vi "get data test.vi"() -> ()   [LabVIEW 2014]
uses:
  Robot Global Data.vi
panel:
  out "unsigned byte array":u8[](array[numeric])
  out "Bytes at Port":u32
  in  "Numeric 4":i32
  in  "milliseconds to wait 2":u32
  in  "milliseconds to wait":u32
  out "Received Data 7":u8[][](array[numeric])
  out "Received Data 6":u8[][](array[numeric])
  in  "write and read":bool
  in  "Numeric 3":i32
  out "Received Data 5":u8[][](array[numeric])
  in  "Numeric 2":i32
  in  "read forloop":bool=TRUE
  out "Received Data 4":u8[](array[numeric])
  in  "array input":bool
  in  "for loop":bool
  out "Received Data 3":u8[][](array[numeric])
  in  "Numeric":i32
  out "Received Data 2":u8[](array[numeric])
  out "distance 2":fxp<+/-,32,16>[](array[numeric])
  out "Received Data":u8[](array[numeric])
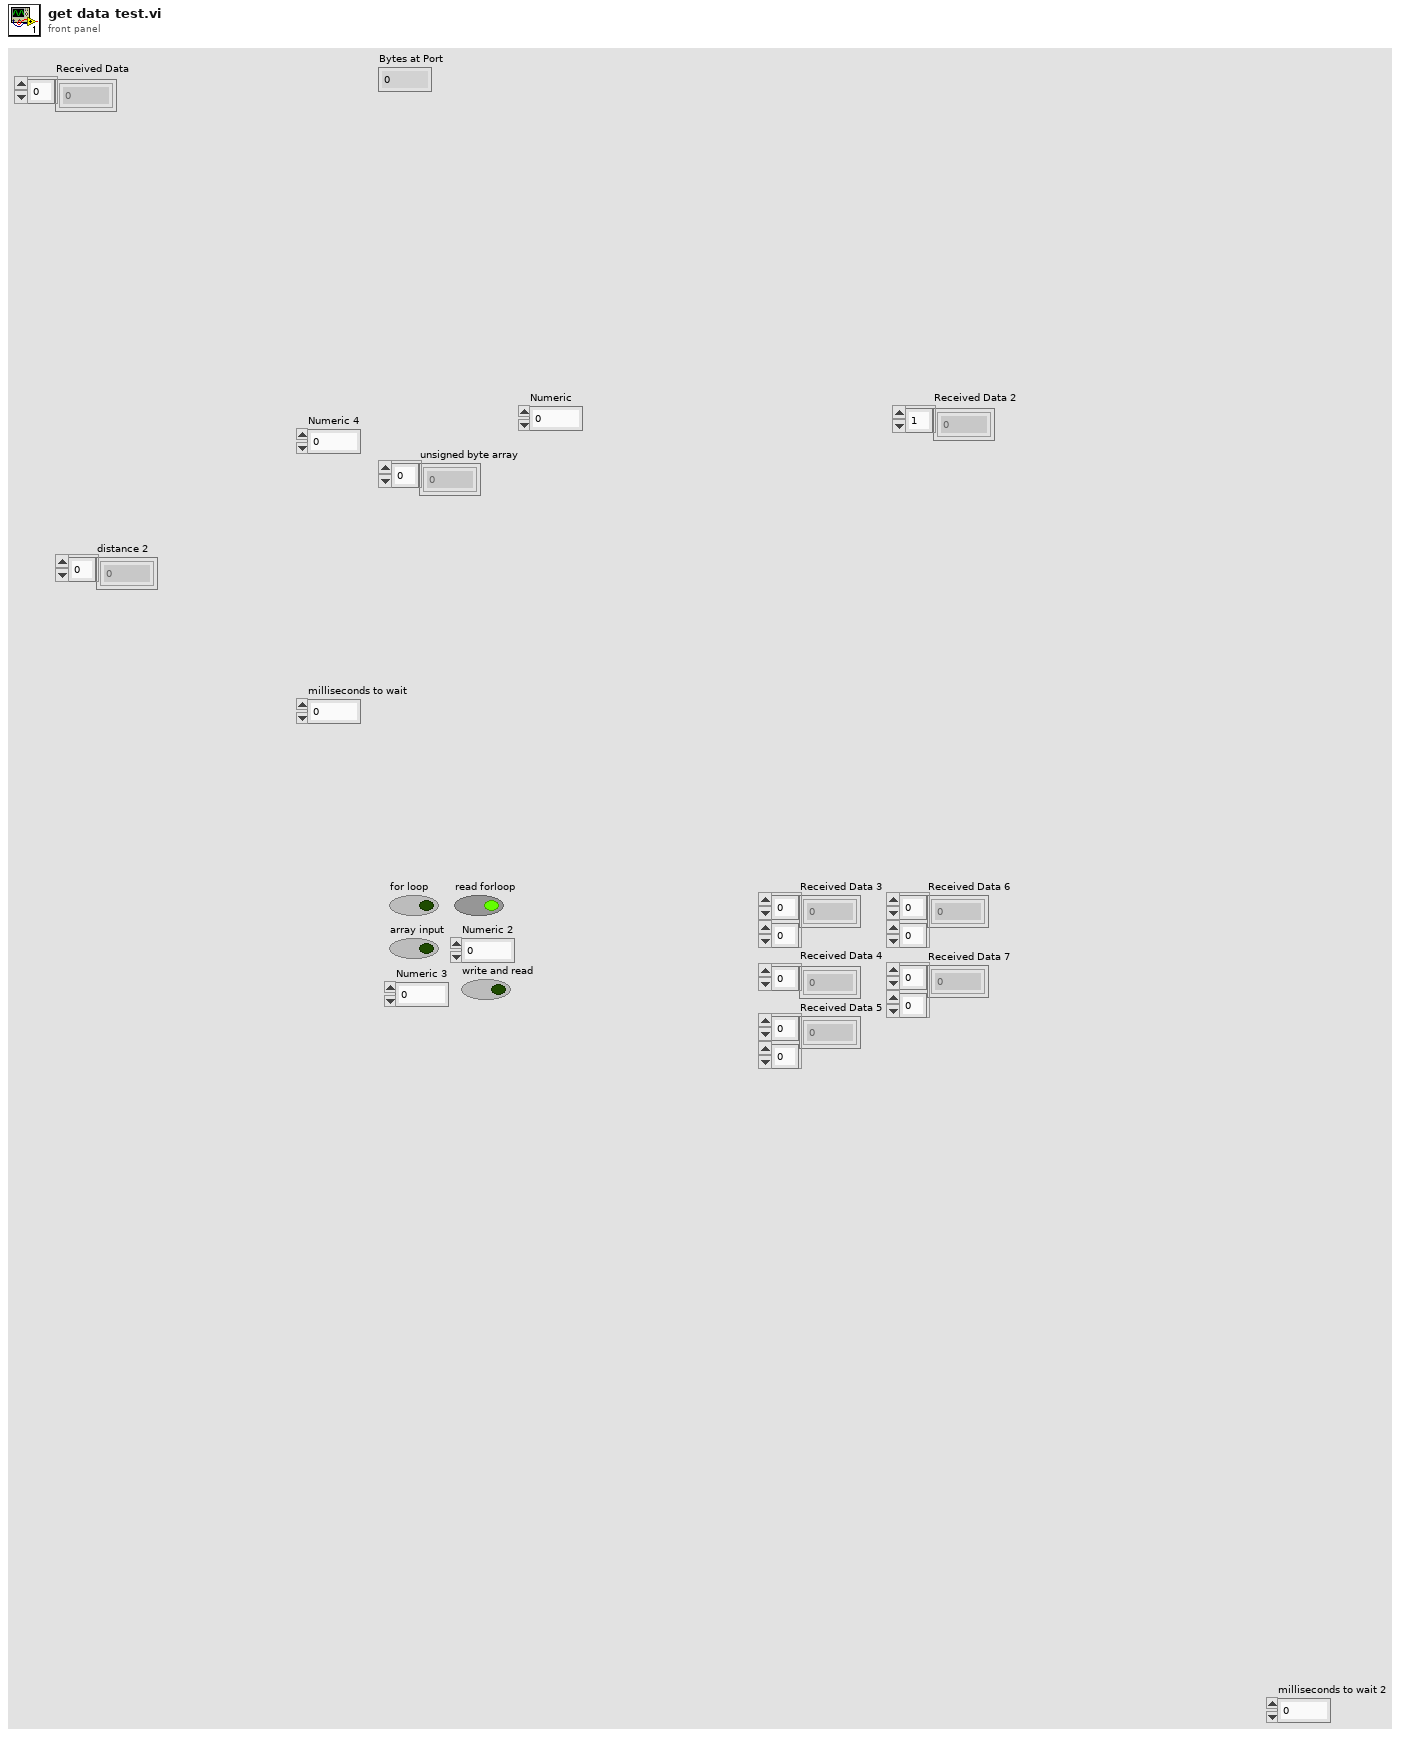
[diagram p1: front panel]
types:
  T1 = typedef "WPI_SPIDevRef.ctl" = cluster{"DevStatus":errorcluster, "Handle":i32, "Controller":T2, "SPI Bus":T3}
  T2 = typedef "FPGA_TypedefDigitalModule.ctl" = enum16{"Controller 1"}
  T3 = typedef "spi_bus.ctl" = enum16{"SPI On-Board, CS0", "SPI On-Board, CS1", "SPI On-Board, CS2", "SPI On-Board, CS3", "SPI MXP", "Invalid"}
  T4 = typedef "WPI_SerialPortRef.ctl" = cluster{"DevStatus":errorcluster, "Serial Port Name":refnum<visa-resource-name>}
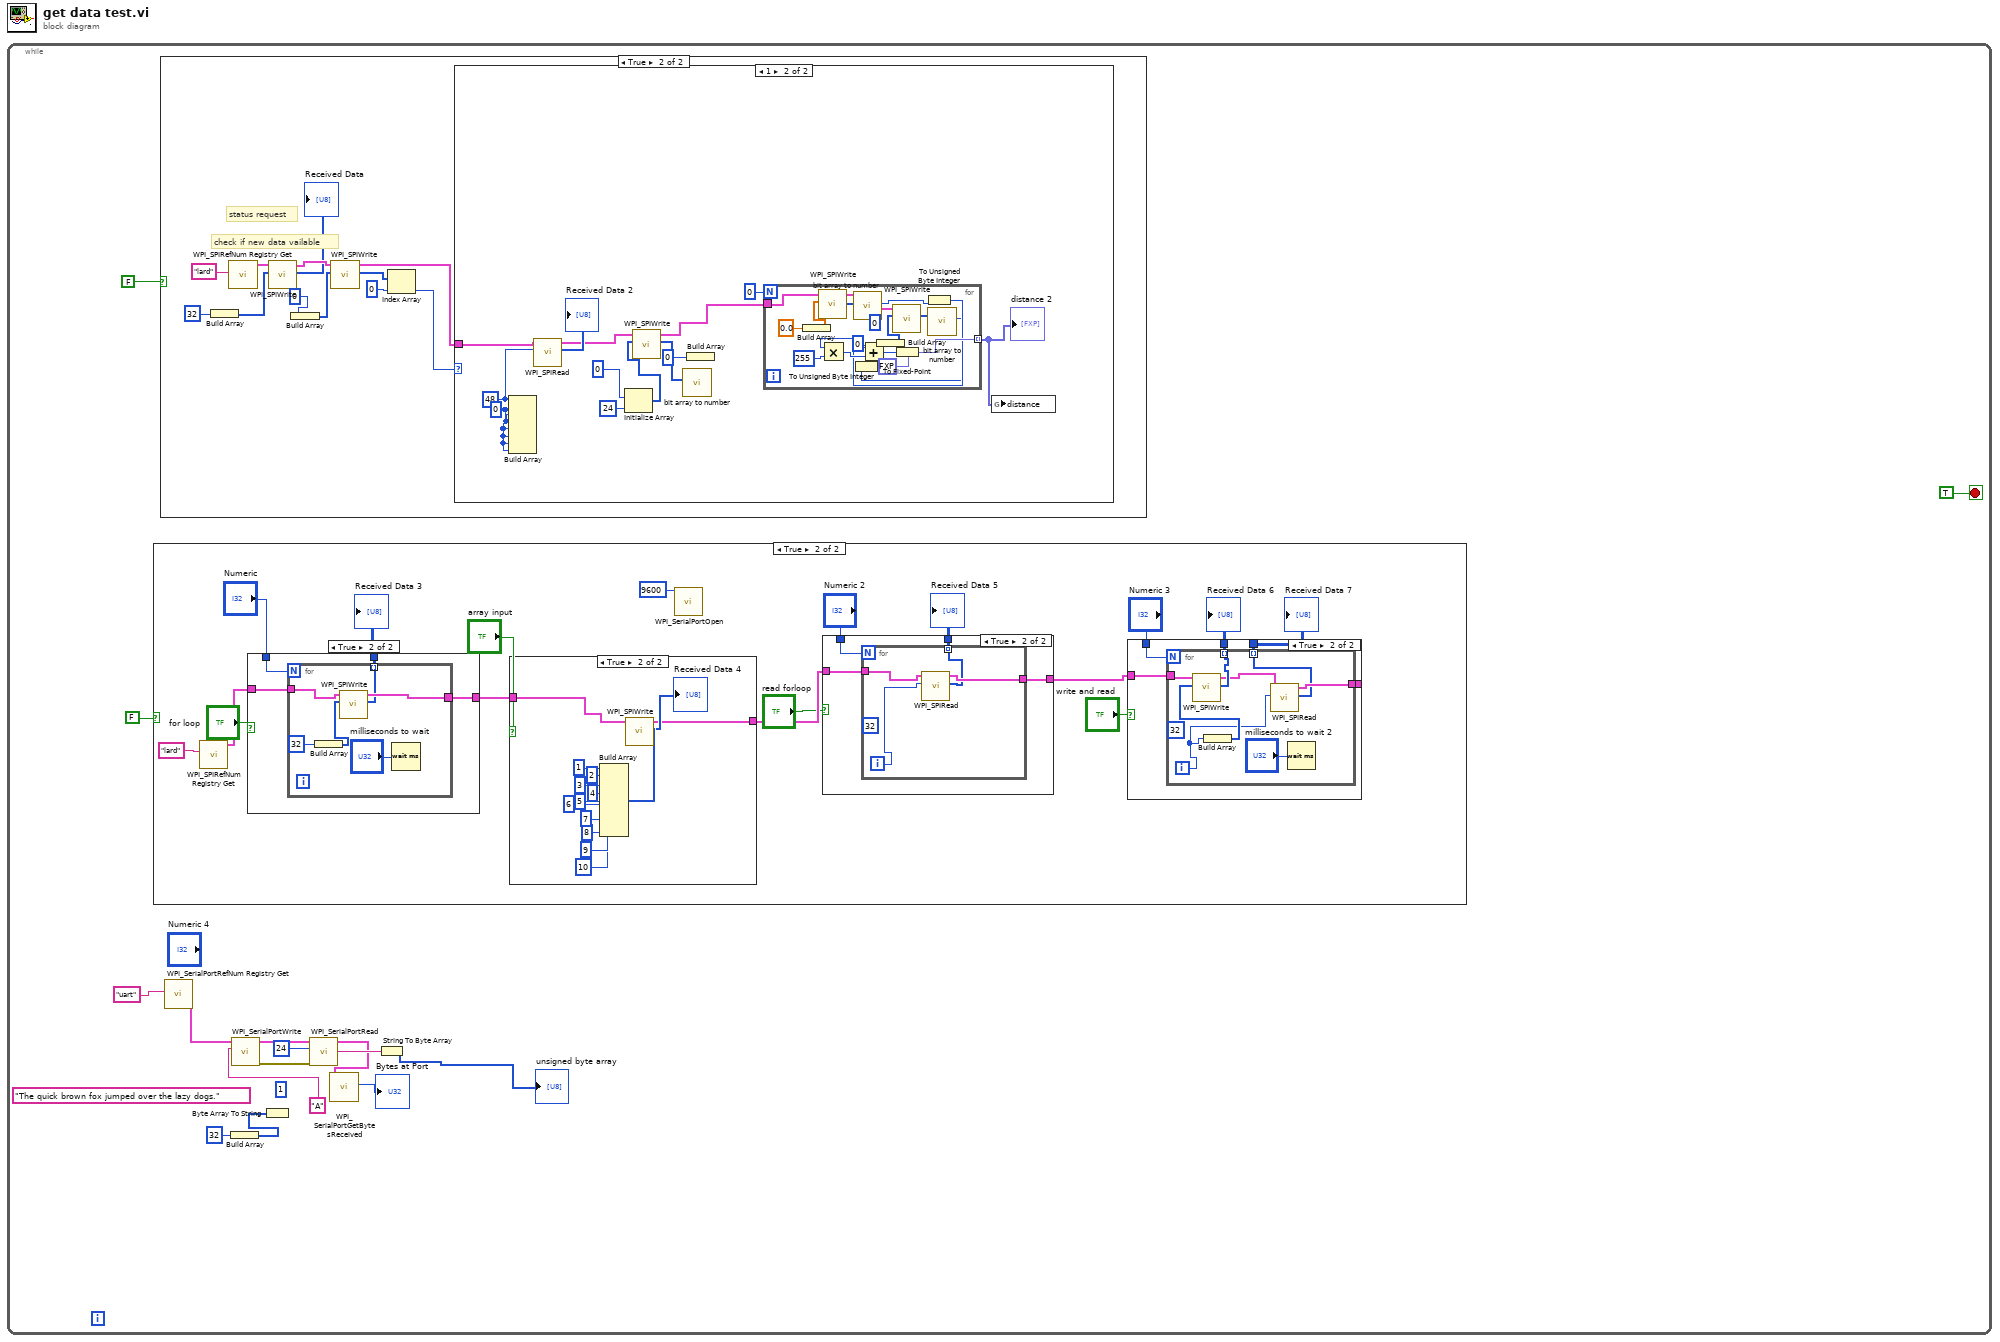
[diagram p0: block diagram]
diagram:
  n1 = while {
    stop <- TRUE stop-if-true
    (unwired) "The quick brown fox jumped over the lazy dogs." ("Buffer")
    (unwired) u32 1 ("Num Bytes to Read")
    n2 = case shown="True" FALSE {
      frame False {
      }
      frame True {
        n3 = call <vilib>:"WPI_SPIRefNum Registry Get.vi"("refnum name"="lard") -> ("SPIDevRef"=w31:T1)  [unwired: 9 in, 1 out]
        n4 = case shown="True" "for loop" {
          tunnel: w31 -> [w71 w75]
          tunnel: "Numeric" -> [_ w74]
          tunnel: [_ w73] -> w29
          tunnel: [w71 w72] -> w26
          frame False {
          }
          frame True {
            n5 = for {
              N: w74 -> [_]
              tunnel: w75 -> [w80]
              tunnel: [w78] -> w73 mode=indexing
              tunnel: [w79] -> w72
              n6 = Build Array(u8 32) -> (w77:u8[])
              n7 = call <vilib>:"WPI_SPIWrite.vi"("Data To Send"=w77, "SPIDevRef"=w80) -> ("Received Data"=w78:u8[], "SPIDevRef"=w79:T1)  [unwired: 1 in, 7 out]
              n8 = Wait (ms)(milliseconds to wait="milliseconds to wait") -> ()  [unwired: 1 out]
            }
          }
        }
        "Received Data 3" <- w29
        n9 = case shown="True" "array input" {
          tunnel: w26 -> [w56 w67]
          tunnel: [w56 w61] -> w25
          frame False {
          }
          frame True {
            n10 = Build Array(1, 2 ("element"), 3 ("element"), 4 ("element"), 5 ("element"), 6 ("element"), 7 ("element"), 8 ("element"), 9 ("element"), 10 ("element")) -> (w70:i32[])
            n11 = call <vilib>:"WPI_SPIWrite.vi"("Data To Send"=w70, "SPIDevRef"=w67) -> ("Received Data"=→"Received Data 4":u8[], "SPIDevRef"=w61:T1)  [unwired: 7 in, 1 out]
          }
        }
        n12 = call <vilib>:"WPI_SerialPortOpen.vi"("Baud Rate"=u32 9600) -> ()  [unwired: 13 in, 2 out]
        n13 = case shown="True" "read forloop" {
          tunnel: w25 -> [w47 w51]
          tunnel: "Numeric 2" -> [_ w50]
          tunnel: [_ w49] -> w22
          tunnel: [w47 w48] -> w21
          frame False {
          }
          frame True {
            n14 = for {
              N: w50 -> [_]
              tunnel: w51 -> [w55]
              tunnel: [w53] -> w49 mode=indexing
              tunnel: [w54] -> w48
              i -> [w52]
              (unwired) 32
              n15 = call <vilib>:"WPI_SPIRead.vi"("Num to Read"=w52, "SPIDevRef"=w55) -> ("Received Data"=w53:u8[], "SPIDevRef"=w54:T1)  [unwired: 1 in, 7 out]
            }
          }
        }
        "Received Data 5" <- w22
        n16 = case shown="True" "write and read" {
          tunnel: w21 -> [w33 w38]
          tunnel: "Numeric 3" -> [_ w37]
          tunnel: [_ w36] -> w17
          tunnel: [w33 w35] -> _
          tunnel: [_ w34] -> w18
          frame False {
          }
          frame True {
            n17 = for {
              N: w37 -> [_]
              tunnel: w38 -> [w46]
              tunnel: [w40] -> w36 mode=indexing
              tunnel: [w42] -> w35
              tunnel: [w45] -> w34 mode=indexing
              i -> [w41]
              (unwired) 32
              n18 = Build Array(w41) -> (w44:i32[])
              n19 = call <vilib>:"WPI_SPIWrite.vi"("Data To Send"=w44, "SPIDevRef"=w46) -> ("Received Data"=w45:u8[], "SPIDevRef"=w43:T1)  [unwired: 1 in, 7 out]
              n20 = call <vilib>:"WPI_SPIRead.vi"("Num to Read"=w41, "SPIDevRef"=w43) -> ("Received Data"=w40:u8[], "SPIDevRef"=w42:T1)  [unwired: 1 in, 7 out]
              n21 = Wait (ms)(milliseconds to wait="milliseconds to wait 2") -> ()  [unwired: 1 out]
            }
          }
        }
        "Received Data 6" <- w18
        "Received Data 7" <- w17
      }
    }
    n22 = case shown="True" FALSE {
      frame False {
      }
      frame True {
        # "status request"
        # "check if new data vailable"
        n23 = Build Array(32) -> (w88:i32[])
        n24 = call <vilib>:"WPI_SPIRefNum Registry Get.vi"("refnum name"="lard") -> ("SPIDevRef"=w84:T1)  [unwired: 9 in, 1 out]
        n25 = call <vilib>:"WPI_SPIWrite.vi"("Data To Send"=w88, "SPIDevRef"=w84) -> ("Received Data"=→"Received Data":u8[], "SPIDevRef"=w91:T1)  [unwired: 7 in, 1 out]
        n26 = Build Array(0 ("Num to Read")) -> (w93:i32[])
        n27 = call <vilib>:"WPI_SPIWrite.vi"("Data To Send"=w93, "SPIDevRef"=w91) -> ("Received Data"=w92:u8[], "SPIDevRef"=w83:T1)  [unwired: 7 in, 1 out]
        n28 = Index Array(array=w92, index=0) -> (element=w82:u8)
        n29 = case shown="1" w82 {
          tunnel: w83 -> [_ w96]
          frame 0, Default {
          }
          frame 1 {
            w98 = 0 ("element")
            w94 = 48
            n30 = Build Array(w94, w98, w98, w98, w98, w98, w98, w98) -> ()  [unwired: 1 out]
            n31 = call <vilib>:"WPI_SPIRead.vi"("Num to Read"=w94, "SPIDevRef"=w96) -> ("Received Data"=→"Received Data 2":u8[], "SPIDevRef"=w95:T1)  [unwired: 7 in, 1 out]
            n32 = Initialize Array(0 ("Num to Read"), 24 ("dimension size")) -> (w101:i32[])
            n33 = call <vilib>:"WPI_SPIWrite.vi"("Data To Send"=w101, "SPIDevRef"=w95) -> ("Received Data"=w105:u8[], "SPIDevRef"=w100:T1)  [unwired: 7 in, 1 out]
            n34 = call "bit array to number.vi"("bit array"=w105) -> ()  [unwired: 10 in, 1 out]
            n35 = Build Array(0 ("Num to Read")) -> ()  [unwired: 1 out]
            n36 = for {
              N: 0 -> [_]
              tunnel: [w123] -> w106 mode=indexing
              tunnel: w100 -> [w109]
              (unwired) 0 ("Num to Read")
              n37 = Build Array(0.0 ("element")) -> (w108:dbl[])
              n38 = call <vilib>:"WPI_SPIWrite.vi"("Data To Send"=w108, "SPIDevRef"=w109) -> ("Received Data"=w114:u8[], "SPIDevRef"=w111:T1)  [unwired: 7 in, 1 out]
              n39 = call "bit array to number.vi"("bit array"=w114) -> ("Numeric"=w118:i32)  [unwired: 10 in]
              n40 = Build Array(0 ("Num to Read")) -> (w112:i32[])
              n41 = call <vilib>:"WPI_SPIWrite.vi"("Data To Send"=w112, "SPIDevRef"=w111) -> ("Received Data"=w110:u8[])  [unwired: 7 in, 2 out]
              n42 = To Unsigned Byte Integer(number=w118) -> (unsigned 8bit integer=w117:u8)
              n43 = Multiply(x=w117, y=255) -> (x*y=w121:i32)
              n44 = call "bit array to number.vi"("bit array"=w110) -> ("Numeric"=w115:i32)  [unwired: 10 in]
              n45 = To Unsigned Byte Integer(number=w115) -> (unsigned 8bit integer=w116:u8)
              n46 = Add(x=w116, y=w121) -> (x+y=w120:i32)
              n47 = To Fixed-Point(fixed-point type=fxp<+/-,32,16> 8.0, number=w120) -> (fixed-point=w123:fxp<+/-,32,16>)
            }
            "distance 2" <- w106
            n48 = global write "Robot Global Data.vi" "distance"(w106) -> ()
          }
        }
      }
    }
    n49 = call <vilib>:"WPI_SerialPortRefNum Registry Get.vi"("refnum name"="uart") -> ("SerialPortRef"=w11:T4)  [unwired: 9 in, 1 out]
    n50 = Build Array(u8 32 ("element")) -> (w5:u8[])
    n51 = call <vilib>:"WPI_SerialPortWrite.vi"("Buffer"="A", "SerialPortRef"=w11) -> ("error out"=w9:errorcluster, "SerialPortRef"=w8:T4)  [unwired: 7 in, 1 out]
    n52 = Byte Array To String(unsigned byte array=w5) -> ()  [unwired: 1 out]
    n53 = call <vilib>:"WPI_SerialPortRead.vi"("error in (no error)"=w9, "Num Bytes to Read"=u32 24, "SerialPortRef"=w8) -> ("Buffer"=w7:string, "SerialPortRef"=w4:T4)  [unwired: 6 in, 1 out]
    n54 = call <vilib>:"WPI_SerialPortGetBytesReceived.vi"("SerialPortRef"=w4) -> ("Bytes at Port"=→"Bytes at Port":u32)  [unwired: 8 in, 2 out]
    n55 = String To Byte Array(string=w7) -> (unsigned byte array=→"unsigned byte array":u8[])
  }
